vi "S2DS_Unit selection (SubVI).vi"(11 "RC instrument name":string) -> (2 "Base unit":string, 3 "Instrument default prefix":string)   [LabVIEW 2025]
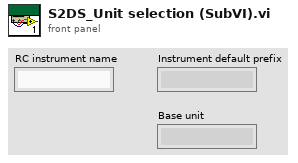
[diagram p1: front panel]
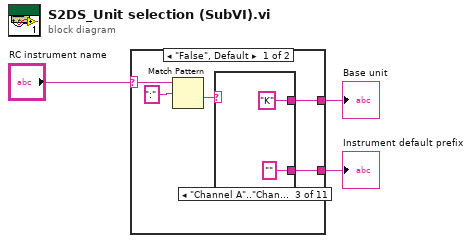
[diagram p0: block diagram]
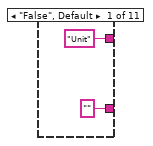
[diagram p2: hidden frame]
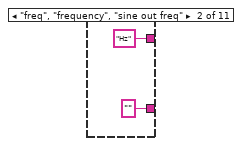
[diagram p3: hidden frame]
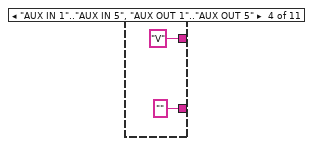
[diagram p4: hidden frame]
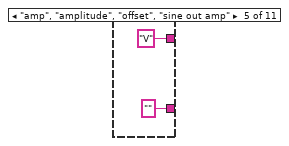
[diagram p5: hidden frame]
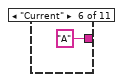
[diagram p6: hidden frame]
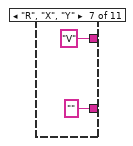
[diagram p7: hidden frame]
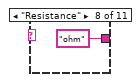
[diagram p8: hidden frame]
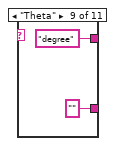
[diagram p9: hidden frame]
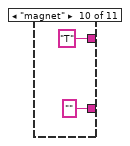
[diagram p10: hidden frame]
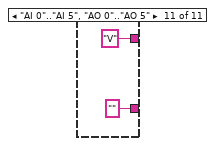
[diagram p11: hidden frame]
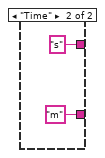
[diagram p12: hidden frame]
diagram:
  n1 = case shown="\"False\", Default" "RC instrument name" {
    selector: "RC instrument name" -> [w7 _]
    tunnel: [w5 "s"] -> w2
    tunnel: [w4 "m"] -> w3
    frame "False", Default {
      n2 = Match Pattern(string=w7, regular expression=":") -> (after substring=w6:string)  [unwired: 1 in, 3 out]
      n3 = case shown="\"Channel A\"..\"Channel E\", \"Temp\", \"temperature\"" w6 {
        tunnel: ["Unit" "Hz" "K" "V" "V" "A" "V" "ohm" "degree" "T" "V"] -> w5
        tunnel: ["" "" "" "" "" _ "" _ "" "" ""] -> w4
        frame "False", Default {
        }
        frame "freq", "frequency", "sine out freq" {
        }
        frame "Channel A".."Channel E", "Temp", "temperature" {
        }
        frame "AUX IN 1".."AUX IN 5", "AUX OUT 1".."AUX OUT 5" {
        }
        frame "amp", "amplitude", "offset", "sine out amp" {
        }
        frame "Current" {
        }
        frame "R", "X", "Y" {
        }
        frame "Resistance" {
        }
        frame "Theta" {
        }
        frame "magnet" {
        }
        frame "AI 0".."AI 5", "AO 0".."AO 5" {
        }
      }
    }
    frame "Time" {
    }
  }
  "Instrument default prefix" <- w3
  "Base unit" <- w2
